vi "Harv_2_9.vi"(0 "HarvSetpoints":dbl[](array[numeric]), 1 "HarvPot":dbl, 3 "Count":i32, 4 "BallAcquired":bool, 5 "FireBallSen":bool, 6 "Fire":bool, 7 "Harvest":bool, 8 "HPButton":bool, 9 "inAuton?":bool, 10 "WinchDown":bool, 11 "AutonMoved":bool, 12 "HarvPivUP":bool, 13 "HarvPivPickupLim":bool) -> (14 "HarvPower":dbl, 15 "HarvRoller":dbl, 16 "AutonReadyToMove":bool, 17 "CountOut":i32, 18 "HarvStart":bool, 19 "HarvCleared":bool)   [LabVIEW 2013]
panel:
  in  "MotorScale":dbl=1.5
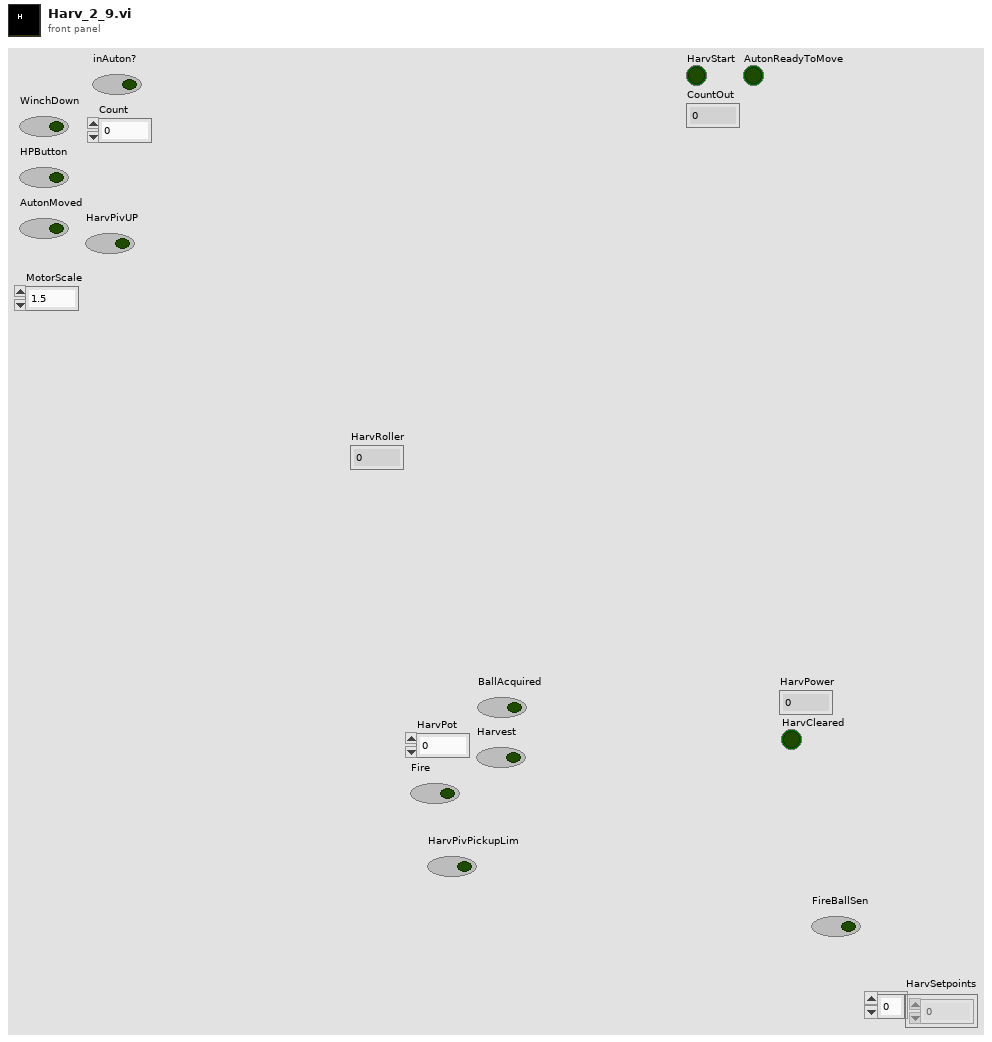
[diagram p1: front panel]
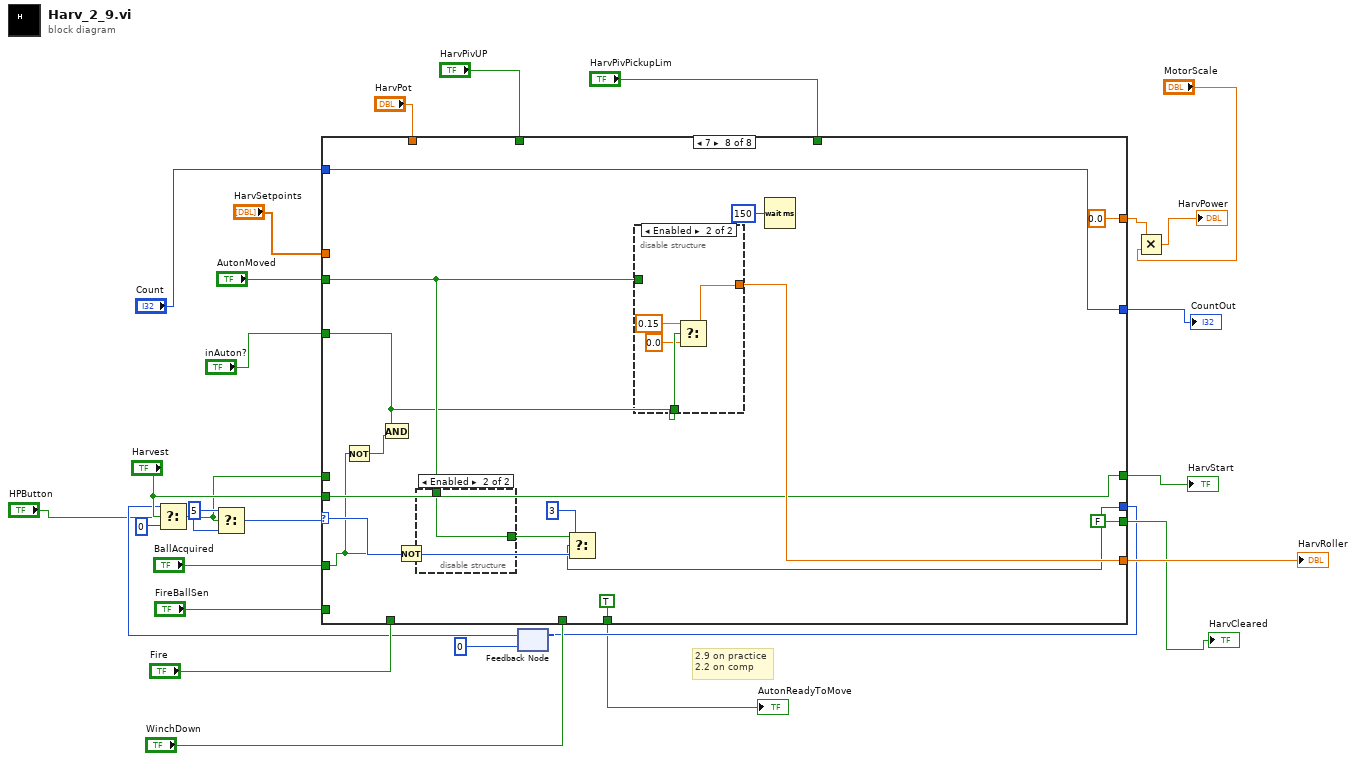
[diagram p0: block diagram]
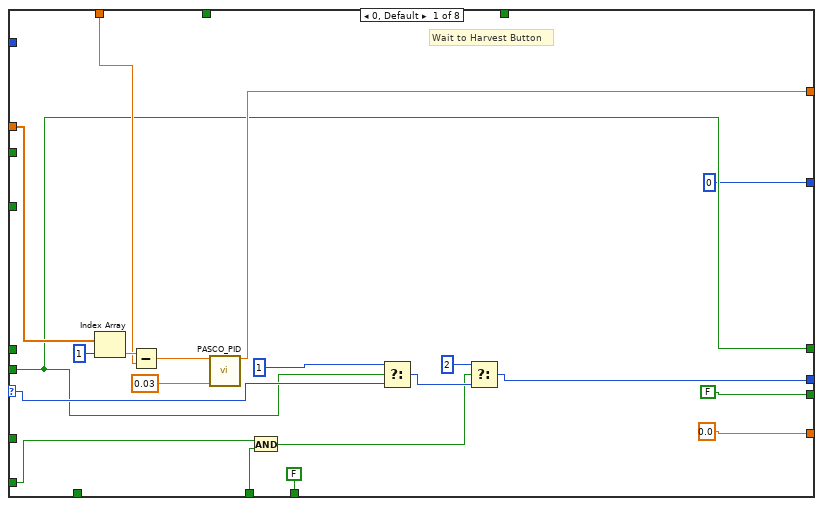
[diagram p2: hidden frame]
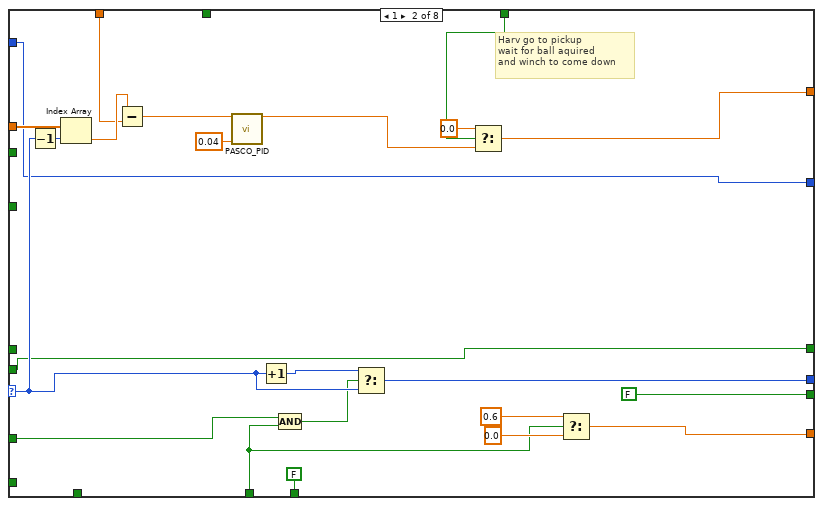
[diagram p3: hidden frame]
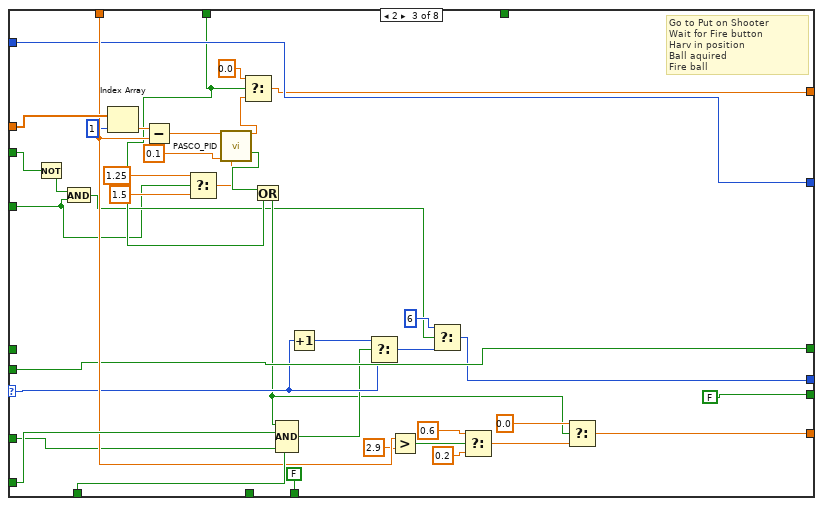
[diagram p4: hidden frame]
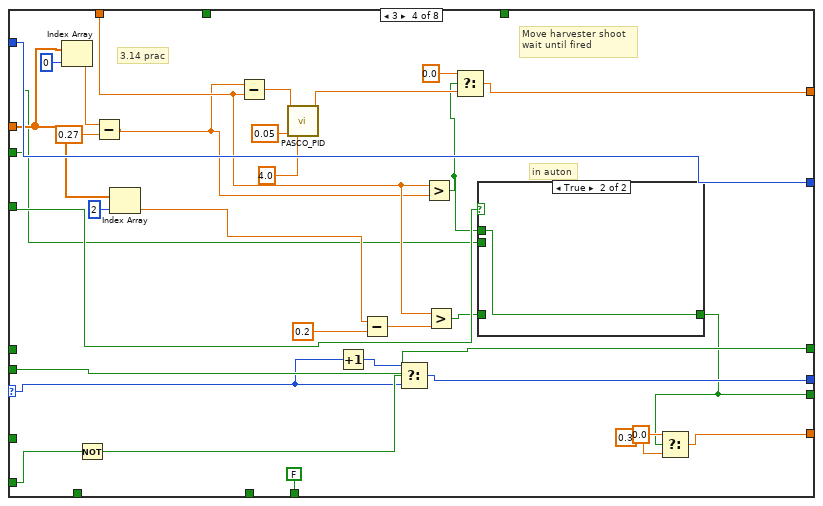
[diagram p5: hidden frame]
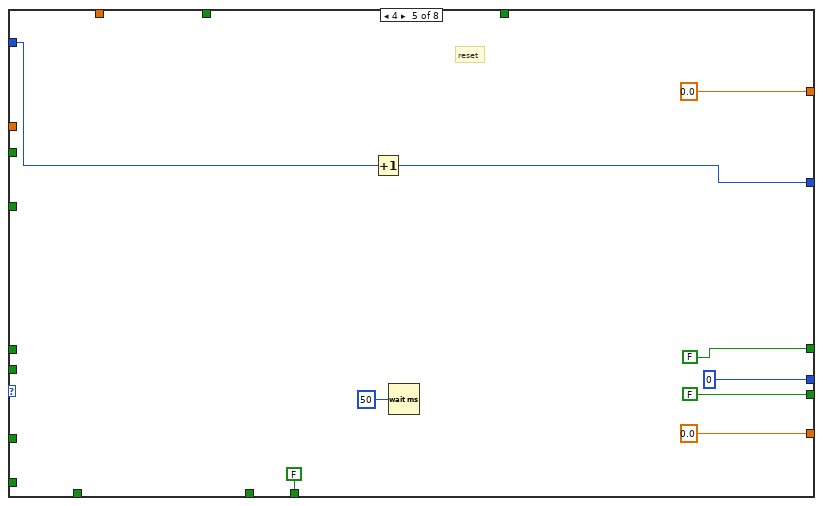
[diagram p7: hidden frame]
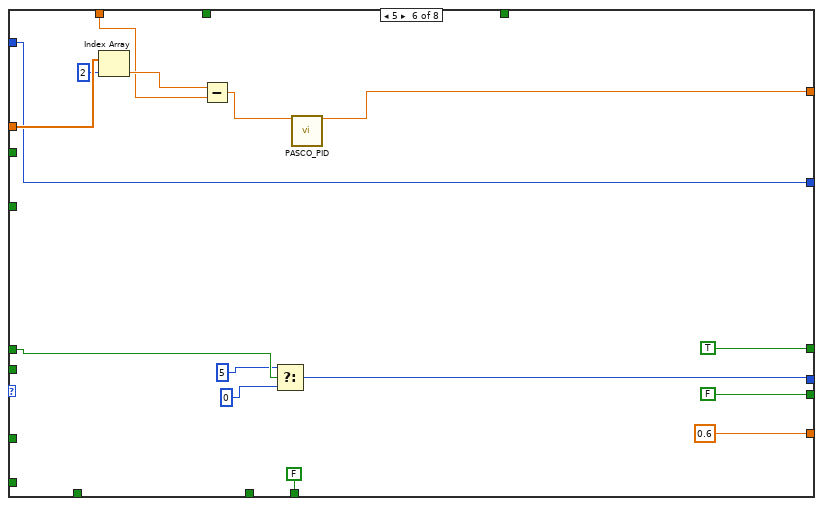
[diagram p8: hidden frame]
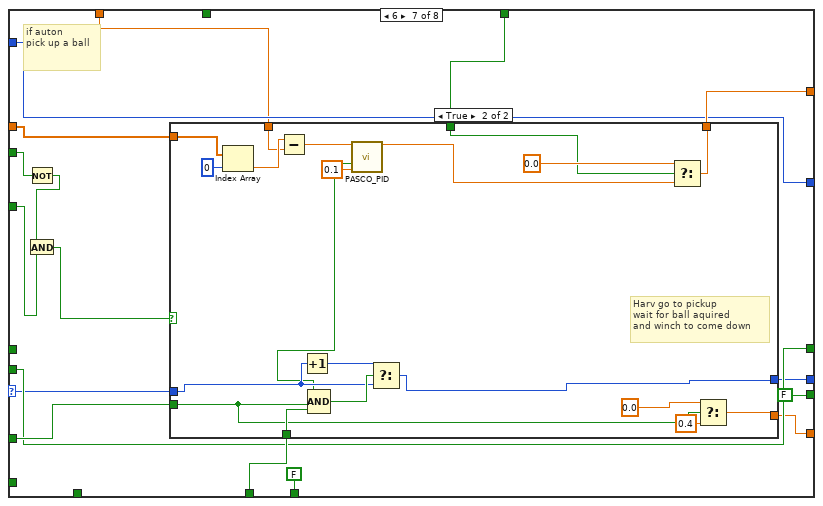
[diagram p9: hidden frame]
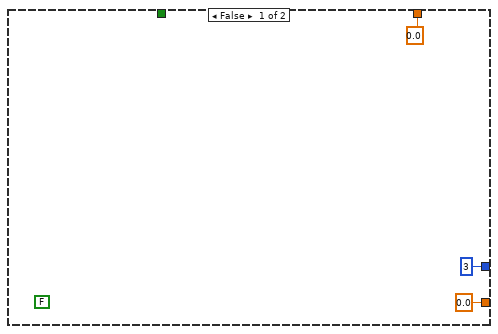
[diagram p10: hidden frame]
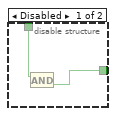
[diagram p11: hidden frame]
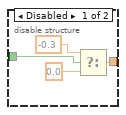
[diagram p12: hidden frame]
diagram:
  # "2.9 on practice\n2.2 on comp"
  n1 = feedback #1(0 ("f")) -> (w21:i32)
  n2 = Select(t=w21, s="Harvest", f=0) -> (s? t:f=w6:i32)
  n3 = Select(t=5, s="HPButton", f=w6) -> (s? t:f=w5:i32)
  n4 = case shown="7" w5 {
    selector: w5 -> [w45 w64 w92 w136 _ _ w177 w218]
    tunnel: "HarvSetpoints" -> [w44 w71 w110 w123 _ w168 w184 _]
    tunnel: "HarvPot" -> [w43 w69 w104 w128 _ w165 w171 _]
    tunnel: [w38 w51 w82 w129 0.0 ("Output") w163 w183 0.0 ("Output")] -> w20
    tunnel: [w35 w66 w84 w141 0 ("t") w158 w178 w217] -> w10
    tunnel: [0.0 ("f") w58 w97 w114 0.0 ("f") 0.6 ("f") w179 w220] -> w26
    tunnel: "BallAcquired" -> [_ w60 w94 _ _ _ w181 w210]
    tunnel: "FireBallSen" -> [w33 _ w107 w139 _ _ _ _]
    tunnel: "Fire" -> [_ _ w106 _ _ _ _ _]
    tunnel: "Harvest" -> [w36 w61 w95 w140 _ _ w180 w219]
    tunnel: [FALSE ("IsThere") FALSE ("IsThere") FALSE ("IsThere") w111 FALSE ("IsThere") FALSE ("IsThere") FALSE ("IsThere") FALSE ("IsThere")] -> w17
    tunnel: "HarvPivPickupLim" -> [_ w53 _ _ _ _ w185 _]
    tunnel: "HarvPivUP" -> [_ _ w87 _ _ _ _ _]
    tunnel: [w36 w61 w95 w140 FALSE ("Harvest") TRUE ("Harvest") w180 w219] -> w14
    tunnel: "WinchDown" -> [w32 w55 _ _ _ _ w182 _]
    tunnel: "inAuton?" -> [_ _ w73 w118 _ _ w172 w209]
    tunnel: [0 ("Count") w54 w91 w135 w147 w162 w176 w222] -> w8
    tunnel: "Count" -> [_ w54 w91 w135 w146 w162 w176 w222]
    tunnel: "HPButton" -> [_ _ _ _ _ w161 _ _]
    tunnel: [FALSE FALSE FALSE FALSE FALSE FALSE FALSE TRUE] -> w2
    tunnel: "AutonMoved" -> [_ _ w79 w115 _ _ w170 w213]
    frame 0, Default {
      # "Wait to Harvest Button"
      n5 = Index Array(array=w44, index=1) -> (element=w46:dbl)
      n6 = Subtract(x=w46, y=w43) -> (x-y=w47:dbl)
      n7 = call "PASCO_PID.vi"("Delta"=w47, "Deadband"=0.03) -> ("Output"=w38:dbl)  [unwired: 12 in, 1 out]
      n8 = And(x=w33, y=w32) -> (x .and. y?=w31:bool)
      n9 = Select(t=1, s=w36, f=w45) -> (s? t:f=w37:i32)
      n10 = Select(t=2, s=w31, f=w37) -> (s? t:f=w35:i32)
    }
    frame 1 {
      # "Harv go to pickup\nwait for ball aquired\nand winch to come down"
      n11 = Decrement(x=w64) -> (x-1=w65:i32)
      n12 = Index Array(array=w71, index=w65) -> (element=w70:dbl)
      n13 = Subtract(x=w70, y=w69) -> (x-y=w68:dbl)
      n14 = call "PASCO_PID.vi"("Delta"=w68, "Deadband"=0.04) -> ("Output"=w52:dbl)  [unwired: 12 in, 1 out]
      n15 = Increment(x=w64) -> (x+1=w67:i32)
      n16 = Compound Arithmetic op=AND(w60, w55) -> (w59:bool)
      n17 = Select(t=w67, s=w59, f=w64) -> (s? t:f=w66:i32)
      n18 = Select(t=0.0, s=w53, f=w52) -> (s? t:f=w51:dbl)
      n19 = Select(t=0.6, s=w55, f=0.0) -> (s? t:f=w58:dbl)
    }
    frame 2 {
      # "Go to Put on Shooter\nWait for Fire button\nHarv in position\nBall aquired \nFire ball"
      n20 = Not(x=w79) -> (.not. x?=w78:bool)
      n21 = And(x=w78, y=w73) -> (x .and. y?=w77:bool)
      n22 = Index Array(array=w110, index=1) -> (element=w109:dbl)
      n23 = Subtract(x=w109, y=w104) -> (x-y=w108:dbl)
      n24 = Select(t=1.25, s=w73, f=1.5) -> (s? t:f=w76:dbl)
      n25 = call "PASCO_PID.vi"("Delta"=w108, "Deadband"=0.1, "P Gain"=w76) -> ("Output"=w90:dbl, "IsThere"=w88:bool)  [unwired: 11 in]
      n26 = Select(t=0.0, s=w87, f=w90) -> (s? t:f=w82:dbl)
      n27 = Or(x=w88, y=w87) -> (x .or. y?=w80:bool)
      n28 = Compound Arithmetic op=AND(w80, w107, w106, w94) -> (w81:bool)
      n29 = Increment(x=w92) -> (x+1=w93:i32)
      n30 = Select(t=w93, s=w81, f=w92) -> (s? t:f=w85:i32)
      n31 = Greater?(x=w104, y=2.9) -> (0:w102:bool)
      n32 = Select(t=6, s=w77, f=w85) -> (s? t:f=w84:i32)
      n33 = Select(t=0.6, s=w102, f=0.2) -> (s? t:f=w98:dbl)
      n34 = Select(t=0.0, s=w80, f=w98) -> (s? t:f=w97:dbl)
    }
    frame 3 {
      # "in auton"
      # "3.14 prac"
      # "Move harvester shoot\nwait until fired"
      n35 = Index Array(array=w123, index=0) -> (element=w122:dbl)
      n36 = Not(x=w139) -> (.not. x?=w138:bool)
      n37 = Subtract(x=w122, y=0.27) -> (x-y=w121:dbl)
      n38 = Index Array(array=w123, index=2) -> (element=w126:dbl)
      n39 = Subtract(x=w121, y=w128) -> (x-y=w134:dbl)
      n40 = call "PASCO_PID.vi"("Delta"=w134, "Deadband"=0.05, "P Gain"=4.0) -> ("Output"=w130:dbl)  [unwired: 11 in, 1 out]
      n41 = Increment(x=w136) -> (x+1=w137:i32)
      n42 = Subtract(x=w126, y=0.2) -> (x-y=w127:dbl)
      n43 = Select(t=w137, s=w138, f=w136) -> (s? t:f=w141:i32)
      n44 = Greater?(x=w128, y=w121) -> (0:w116:bool)
      n45 = Greater?(x=w128, y=w127) -> (0:w117:bool)
      n46 = Select(t=0.0, s=w116, f=w130) -> (s? t:f=w129:dbl)
      n47 = case shown="True" w118 {
        tunnel: [w143 w144] -> w111
        tunnel: w117 -> [w143 _]
        tunnel: w116 -> [_ w144]
        tunnel: w115 -> [_ _]
        frame False {
        }
        frame True {
        }
      }
      n48 = Select(t=0.0, s=w111, f=0.3) -> (s? t:f=w114:dbl)
    }
    frame 4 {
      # "reset"
      n49 = Increment(x=w146) -> (x+1=w147:i32)
      n50 = Wait (ms)(milliseconds to wait=u32 50) -> ()  [unwired: 1 out]
    }
    frame 5 {
      n51 = Index Array(array=w168, index=2) -> (element=w166:dbl)
      n52 = Subtract(x=w166, y=w165) -> (x-y=w164:dbl)
      n53 = Select(t=5 ("index"), s=w161, f=0 ("index")) -> (s? t:f=w158:i32)
      n54 = call "PASCO_PID.vi"("Delta"=w164) -> ("Output"=w163:dbl)  [unwired: 13 in, 1 out]
    }
    frame 6 {
      # "if auton \npick up a ball"
      n55 = Not(x=w170) -> (.not. x?=w169:bool)
      n56 = And(x=w169, y=w172) -> (x .and. y?=w173:bool)
      n57 = case shown="True" w173 {
        tunnel: w185 -> [_ w204]
        tunnel: w184 -> [_ w203]
        tunnel: [0.0 ("Output") w201] -> w183
        tunnel: w182 -> [_ w200]
        tunnel: w181 -> [_ w198]
        tunnel: [0.0 ("f") w199] -> w179
        tunnel: [3 w194] -> w178
        tunnel: w177 -> [_ w192]
        tunnel: w171 -> [_ w190]
        frame False {
          (unwired) FALSE
        }
        frame True {
          # "Harv go to pickup\nwait for ball aquired\nand winch to come down"
          n58 = Index Array(array=w203, index=0) -> (element=w191:dbl)
          n59 = Subtract(x=w191, y=w190) -> (x-y=w205:dbl)
          n60 = Increment(x=w192) -> (x+1=w193:i32)
          n61 = call "PASCO_PID.vi"("Delta"=w205, "Deadband"=0.1) -> ("Output"=w207:dbl, "IsThere"=w189:bool)  [unwired: 12 in]
          n62 = Compound Arithmetic op=AND(w189, w198, w200) -> (w195:bool)
          n63 = Select(t=w193, s=w195, f=w192) -> (s? t:f=w194:i32)
          n64 = Select(t=0.0, s=w204, f=w207) -> (s? t:f=w201:dbl)
          n65 = Select(t=0.0, s=w198, f=0.4) -> (s? t:f=w199:dbl)
        }
      }
    }
    frame 7 {
      n66 = Not(x=w210) -> (.not. x?=w211:bool)
      n67 = And(x=w209, y=w211) -> ()  [unwired: 1 out]
      n68 = Not(x=w210) -> ()  [unwired: 1 out]
      n69 = disable-structure shown="Enabled" {
        disable-tunnel: w213 -> [w226 w227]
        disable-tunnel: [w225 w227] -> w212
        frame Disabled {
          n70 = And(x=w226, y=w225) -> (x .and. y?=w224:bool)
        }
        frame Enabled {
        }
      }
      n71 = Select(t=3, s=w212, f=w218) -> (s? t:f=w217:i32)
      n72 = disable-structure shown="Enabled" {
        disable-tunnel: [w231 w233] -> w220
        disable-tunnel: w213 -> [w228 _]
        disable-tunnel: w209 -> [_ w235]
        frame Disabled {
          n73 = Select(t=-0.3, s=w228, f=0.0) -> (s? t:f=w231:dbl)
        }
        frame Enabled {
          n74 = Select(t=0.15, s=w235, f=0.0) -> (s? t:f=w233:dbl)
        }
      }
      n75 = Wait (ms)(milliseconds to wait=u32 150) -> ()  [unwired: 1 out]
    }
  }
  "HarvRoller" <- w26
  "HarvCleared" <- w17
  "HarvStart" <- w14
  "CountOut" <- w8
  "AutonReadyToMove" <- w2
  n76 = feedback-in #1(w10) -> ()
  n77 = Multiply(x=w20, y="MotorScale") -> (x*y=→"HarvPower":dbl)
